vi "TestUARTTX.vi"() -> ()   [LabVIEW 2024]
uses:
  f982160e-50d4-41ff-871f-d68aa1408b64.vi
  Driver/CTIPicoVISA.lvlib
panel:
  out "Data 2":string
  in  "Len (LineTerm)":u8
  in  "UART Connector":enum16{"UART0", "UART1"}(ring)
  out "Identity":T1
  in  "Data":string
  in  "Term Char (None)":string
  in  "Baud":u32=115200
  in  "VISA resource name in":refnum<visa-resource-name>
  in  "stop":bool
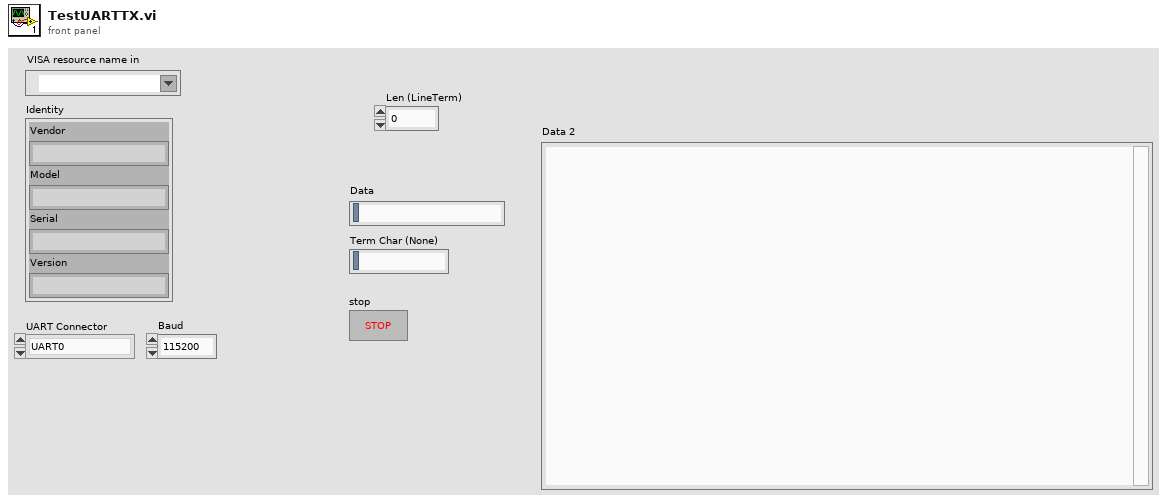
[diagram p1: front panel]
types:
  T1 = cluster{"Vendor":string, "Model":string, "Serial":string, "Version":string}
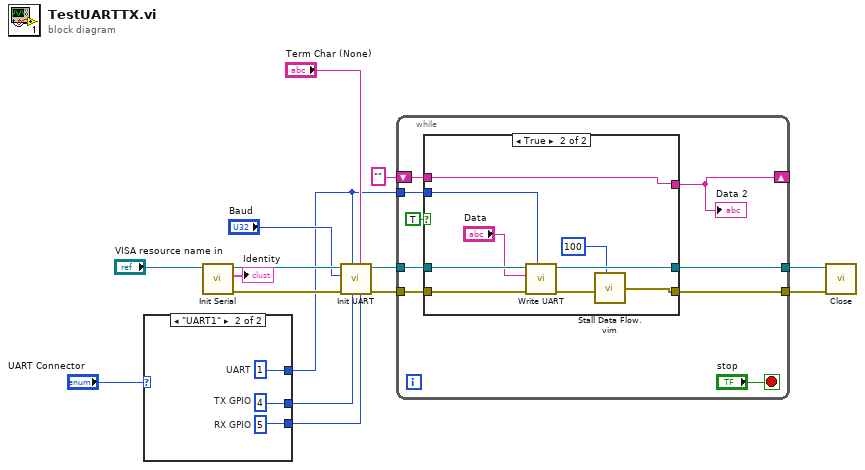
[diagram p0: block diagram]
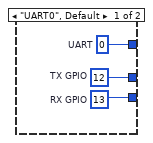
[diagram p2: hidden frame]
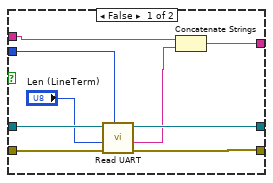
[diagram p3: hidden frame]
diagram:
  n1 = case shown="\"UART1\"" "UART Connector" {
    tunnel: [w18 w19] -> w8
    tunnel: [w17 w20] -> w7
    tunnel: [w16 w21] -> w6
    frame "UART0", Default {
      w17 = u8 13  # RX GPIO
      w18 = u8 12  # TX GPIO
      w16 = u8 0  # UART
    }
    frame "UART1" {
      w20 = u8 5  # RX GPIO
      w19 = u8 4  # TX GPIO
      w21 = u8 1  # UART
    }
  }
  n2 = call "Init Serial.vi"("VISA resource name in"="VISA resource name in") -> ("error out"=w13:errorcluster, "Identity"=→"Identity":T1, "VISA resource name Out"=w14:refnum<visa-resource-name>)  [unwired: 8 in]
  n3 = call "Init UART.vi"("RX GPIO"=w7, "Term Char (None)"="Term Char (None)", "TX GPIO"=w8, "UART"=w6, "error in (no error)"=w13, "Baud"="Baud", "VISA resource name in"=w14) -> ("error out"=w10:errorcluster, "VISA resource name"=w11:refnum<visa-resource-name>)  [unwired: 3 in]
  n4 = while {
    tunnel: w11 -> [w29]
    tunnel: w10 -> [w27]
    tunnel: w6 -> [w28]
    tunnel: [w23] -> w5
    tunnel: [w26] -> w4
    shift-right: [w22] -> _
    shift-left: "" -> [w24]
    stop <- "stop" stop-if-true
    n5 = case shown="True" TRUE {
      tunnel: w29 -> [w39 w48]
      tunnel: w28 -> [w37 w47]
      tunnel: w27 -> [w38 w46]
      tunnel: [w31 w41] -> w23
      tunnel: [w36 w44] -> w26
      tunnel: w24 -> [w34 w43]
      tunnel: [w33 w43] -> w22
      frame False {
        n6 = call "Read UART.vi"("UART"=w37, "error in (no error)"=w38, "Len (LineTerm)"="Len (LineTerm)", "VISA resource name in"=w39) -> ("error out"=w31:errorcluster, "Data"=w32:string, "VISA resource name"=w36:refnum<visa-resource-name>)  [unwired: 5 in]
        n7 = Concatenate Strings(w34, w32) -> (w33:string)
      }
      frame True {
        n8 = call "Write UART.vi"("UART"=w47, "error in (no error)"=w46, "Data"="Data", "VISA resource name in"=w48) -> ("error out"=w42:errorcluster, "VISA resource name"=w44:refnum<visa-resource-name>)  [unwired: 6 in]
        n9 = call "Stall Data Flow.vim"("value in"=w42, "milliseconds to wait"=u32 100) -> ("value out"=w41:errorcluster)  [unwired: 1 out]
      }
    }
    "Data 2" <- w22
  }
  n10 = call "Close.vi"("error in (no error)"=w5, "VISA resource name in"=w4) -> ()  [unwired: 9 in, 1 out]
